vi "CANopenPDOWrite.vi"(2 "Boolean In":bool[](array[boolean]), 3 "Node ID":u8, 4 "error in":errorcluster, 5 "PDO configuration":T1, 6 "DataLength":u8, 7 "FPGA VI Reference In":refnum<k20>) -> (0 "error out":errorcluster, 1 "FPGA VI Reference Out":refnum<k20>)   [LabVIEW 2016]
doc: "This VI updates the configured PDO memory for a particular COB ID. On first call it starts the periodic transmit process."
uses:
  <vilib>/rvi/errors/niLvFpgaAdjustHostInterfaceError.vi
  <vilib>/Utility/error.llb/Error Cluster From Error Code.vi
  <vilib>/rvi/interface/nirviReadWriteControl/nirviReadWriteControl.xnode
  FPGA Bitfiles/EV-MCU_FPGATarget_CANEngine(FPGA)b_eM8Xz3qYJVA.lvbitx
  CAN_Engine(FPGA)_basic.vi
  NiFpgaLv.dll
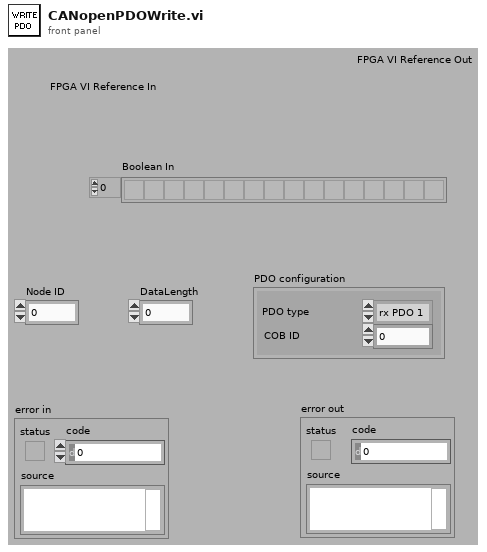
[diagram p1: front panel]
types:
  T1 = cluster{"PDO type":enum8{"rx PDO 1", "rx PDO 2", "rx PDO 3", "rx PDO 4"}, "COB ID":u32}
  T2 = enum8{"rx PDO 1", "rx PDO 2", "rx PDO 3", "rx PDO 4"}
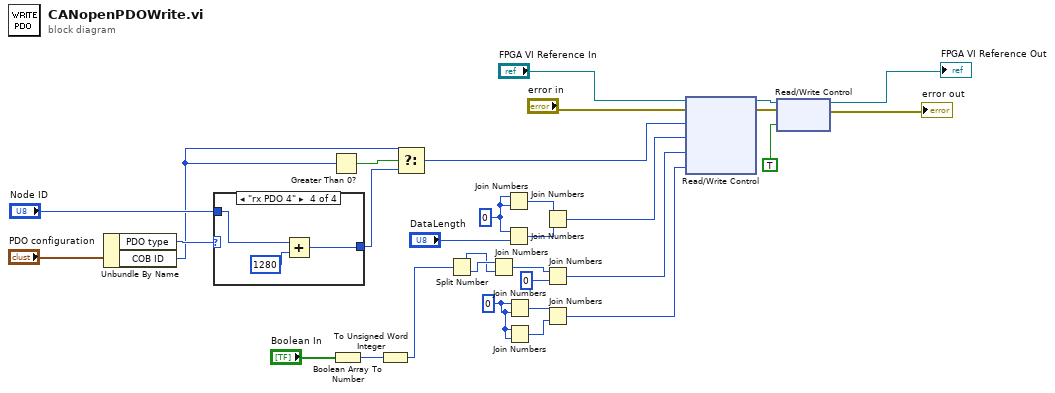
[diagram p0: block diagram]
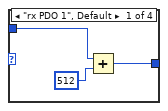
[diagram p2: hidden frame]
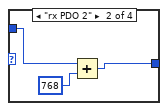
[diagram p3: hidden frame]
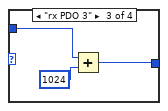
[diagram p4: hidden frame]
diagram:
  w16 = u8 0 ("hi")
  w22 = u8 0 ("lo")
  n1 = Unbundle By Name("PDO configuration") -> ("PDO type"=w30:T2, "COB ID"=w27:u32)
  n2 = case shown="\"rx PDO 4\"" w30 {
    tunnel: "Node ID" -> [w34 w36 w39 w42]
    tunnel: [w32 w35 w38 w41] -> w26
    frame "rx PDO 1", Default {
      n3 = Add(x=w34, y=u32 512) -> (x+y=w32:u32)
    }
    frame "rx PDO 2" {
      n4 = Add(x=w36, y=u32 768) -> (x+y=w35:u32)
    }
    frame "rx PDO 3" {
      n5 = Add(x=w39, y=u32 1024) -> (x+y=w38:u32)
    }
    frame "rx PDO 4" {
      n6 = Add(x=w42, y=u32 1280) -> (x+y=w41:u32)
    }
  }
  n7 = Greater Than 0?(x=w27) -> (x > 0?=w28:bool)
  n8 = Boolean Array To Number(Boolean array="Boolean In") -> (number=w20:u32)
  n9 = To Unsigned Word Integer(number=w20) -> (unsigned 16bit integer=w14:u16)
  n10 = Select(t=w27, s=w28, f=w26) -> (s? t:f=w10:u32)
  n11 = Split Number(x=w14) -> (hi(x)=w12:u8, lo(x)=w13:u8)
  n12 = Join Numbers(hi=w13, lo=w12) -> ((hi.lo)=w15:u16)
  n13 = Join Numbers(hi=w22, lo=w22) -> ((hi.lo)=w24:u16)
  n14 = Join Numbers(hi=w22, lo="DataLength") -> ((hi.lo)=w25:u16)
  n15 = Join Numbers(hi=w16, lo=w16) -> ((hi.lo)=w19:u16)
  n16 = Join Numbers(hi=w16, lo=w16) -> ((hi.lo)=w18:u16)
  n17 = Join Numbers(hi=w24, lo=w25) -> ((hi.lo)=w9:u32)
  n18 = Join Numbers(hi=w15, lo=u16 0) -> ((hi.lo)=w8:u32)
  n19 = Join Numbers(hi=w19, lo=w18) -> ((hi.lo)=w7:u32)
  n20 = xnode "Read/Write Control"("FPGA VI Reference In"="FPGA VI Reference In", "error in"="error in", "U32 Out 3"=w10, "U32 Out 4"=w9, "U32 Out 5"=w8, "U32 Out 6"=w7) -> ("FPGA VI Reference Out"=w6:refnum<k20>, "error out"=w5:errorcluster)
  n21 = xnode "Read/Write Control"("FPGA VI Reference In"=w6, "error in"=w5, "Write"=TRUE) -> ("FPGA VI Reference Out"=→"FPGA VI Reference Out":refnum<k20>, "error out"=→"error out":errorcluster)
